vi "EventLog.Confirm.vi"(8 "error in":errorcluster, 9 "current time":timestamp, 11 "src":T1) -> (0 "error out":errorcluster)   [LabVIEW 2013]
uses:
  EventLog.EventSource.ctl
  Translator/Translator.Message.ctl
  EventLog.EventGui.ctl
  EventLog.EventLevel.ctl
  EventLog.Buffer.Action.ctl
  EventLog.Event.ctl
  Global/ApplicationGlobal.vi
  User/User.Global.vi
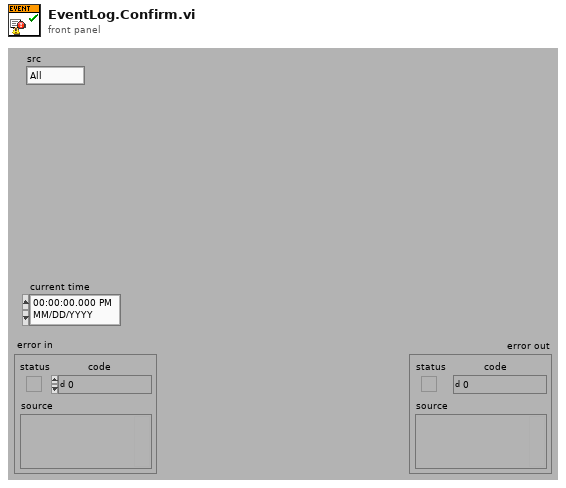
[diagram p1: front panel]
types:
  T1 = typedef "EventLog.EventSource.ctl" = enum16{"All", "Gui", "DB", "Seq", "File", "DIO", "AI", "AO", "IFM", "CPX"}
  T2 = typedef "EventLog.Event.ctl" = cluster{"ts":dbl, "lev":T3, "usr":i32, "src":T1, "msg":T4, "arg":variant[]}
  T3 = typedef "EventLog.EventLevel.ctl" = enum8{"Debug", "Info", "Warning", "Error"}
  T4 = typedef "Translator.Message.ctl" = enum16{"-", "Event confirmed", "Log out", "Log in", "Shutdown", "Cancel", "Start", "Error %d >> %s", "Error %d >> %s >> %s", "Starting %s", "Quitting %s", "User %s level %s added", "User %s level %s deleted", "User %s level %s changed to %s", "Configured", "Initializing", "Quitting", "Loading", "Running", "Stopped", "Do you want to continue?", "Calibration", "Log out?", "System", "All", "IDLE", "Translating...%s", "Not found", "Alarm %s", "Restart is required to translate the application! Do you want to restart the PC?", "Restart cancelled. Be aware that some controls may not be fully translated until you restart the application.", "New version available!", "The software is up-to-date", "PC software will be updated after rebooting the PC. Do you want to reboot now?", "RT software will be updated. Make sure that no process is running. Do you want to reboot RT now?", "Updating RT firmware. Please wait...", "Update failed: %s", "Rebooting...", "Rebooting RT. Please wait...", "RT updated to version %s", "Timeout error during update. Check if RT is working", "Run", "Skip", "Abort", "Please wait...", "Put reference number...", "Folder '%s' is missing", "File '%s' is missing", "File '%s' is broken", "File '%s' is running", "Log file '%s' started", "Step '%s' added to log file", "Log file '%s' ended", "Test steps are missing", "Output %s = %.3f"}
  T5 = typedef "EventLog.Buffer.Action.ctl" = enum16{"init", "re-init", "clear", "set translator", "add", "get"}
  T6 = typedef "EventLog.EventGui.ctl" = cluster{"ts":dbl, "lev":T3, "usr":i32, "src":T1, "msg":T4, "arg":variant[], "msg_str":string}
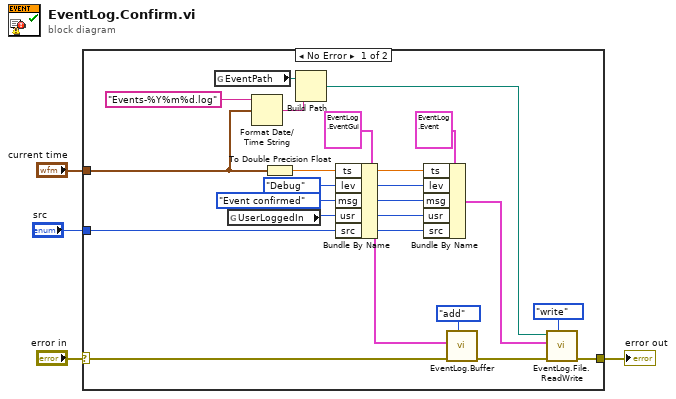
[diagram p0: block diagram]
diagram:
  n1 = case shown="No Error" "error in" {
    selector: "error in" -> [w9 w24]
    tunnel: [w19 w24] -> w4
    tunnel: "current time" -> [w6 _]
    tunnel: "src" -> [w5 _]
    frame No Error {
      w7 = EventLog.EventLevel."Debug" ("lev")
      w16 = Translator.Message."Event confirmed" ("msg")
      n2 = global read "ApplicationGlobal.vi" "EventPath"() -> (w13:path)
      n3 = global read "User.Global.vi" "UserLoggedIn"() -> (w10:i32)
      n4 = Format Date/Time String(time format string (%c)="Events-%Y%m%d.log", seconds (now)=w6) -> (date/time string=w12:string)  [unwired: 1 in]
      n5 = To Double Precision Float(number=w6) -> (double precision float=w17:dbl)
      n6 = Build Path(base path=w13, name or relative path=w12) -> (appended path=w11:path)
      n7 = Bundle By Name(cluster=T6 {"ts"=0.0, "lev"=enum."Debug", "usr"=0, "src"=enum."All", "msg"=enum."Log out", "arg"=[], "msg_str"=""} ("Event in"), "ts"=w17, "lev"=w7, "msg"=w16, "usr"=w10, "src"=w5) -> (w8:T6)
      n8 = Bundle By Name(cluster=T2 {"ts"=0.0, "lev"=enum."Debug", "usr"=0, "src"=enum."All", "msg"=enum."Log out", "arg"=[]} ("event in"), "ts"=w17, "lev"=w7, "msg"=w16, "usr"=w10, "src"=w5) -> (w15:T2)
      n9 = call "EventLog.Buffer.vi"("action (get)"=EventLog.Buffer.Action."add" ("action (read)"), "error in"=w9, "Event in"=w8) -> ("error out"=w20:errorcluster)  [unwired: 5 in, 3 out]
      n10 = call "EventLog.File.ReadWrite.vi"("action (read)"=enum16{"read", "write"}."write", "error in"=w20, "event in"=w15, "file"=w11) -> ("error out"=w19:errorcluster)  [unwired: 3 in, 4 out]
    }
    frame Error {
    }
  }
  "error out" <- w4
